vi "Create RC Connection Monitor.vi"(8 "error in (no error)":errorcluster, 10 "Configure":T1, 11 "RemoteControl in":refnum<class "RemoteControl.v2.lvclass">) -> (0 "error out":errorcluster, 3 "RemoteControl out":refnum<class "RemoteControl.v2.lvclass">)   [LabVIEW 2016, in "RemoteControl.v2.lvclass"]
uses:
  RemoteControl.v2.lvclass
  C:/Program Files (x86)/National Instruments/LabVIEW 2016/vi.lib/JKI/JKI SMO/SMO/SMO.lvclass
  Typedefs/PrivateEvents--RemoteControl.Configure.ctl
  Typedefs/RC Process Type--Enum.ctl
  RemoteControl.v2.lvclass/RemoteControl.v2.ctl
  <vilib>/JKI/JKI SMO/SMO/SMO.lvclass
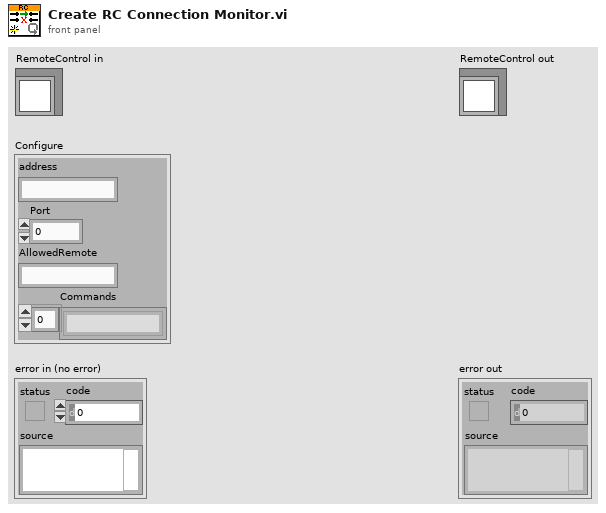
[diagram p1: front panel]
types:
  T1 = typedef "RemoteControl.v2.lvclass/PrivateEvents--RemoteControl.Configure.ctl" = cluster{"address":string, "Port":u16, "AllowedRemote":string, "Commands":string[]}
  T2 = typedef "RemoteControl.v2.lvclass/RC Process Type--Enum.ctl" = enum16{"Connection Monitor", "Server", "Client"}
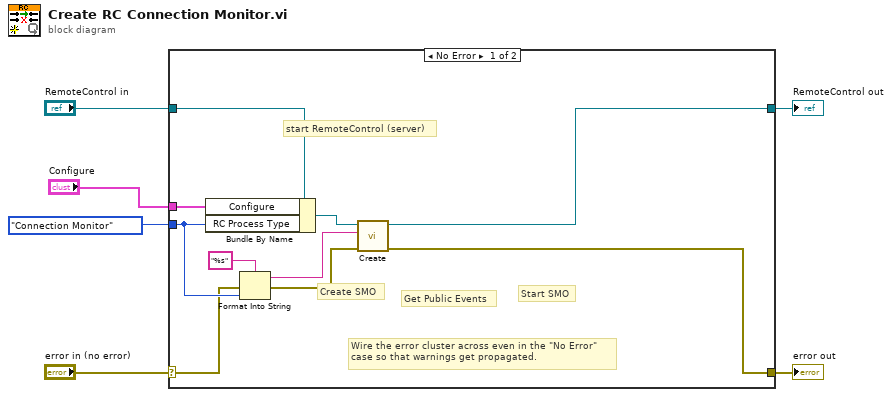
[diagram p0: block diagram]
diagram:
  n1 = case shown="No Error" "error in (no error)" {
    selector: "error in (no error)" -> [w9 w18]
    tunnel: [w8 w18] -> w5
    tunnel: [w7 w17] -> w3
    tunnel: "RemoteControl in" -> [w15 w17]
    tunnel: RC_Process_Type--Enum."Connection Monitor" ("RC Process Type") -> [w13 _]
    tunnel: "Configure" -> [w14 _]
    frame No Error {
      # "start RemoteControl (server)"
      # "Get Public Events"
      # "Start SMO"
      # "Create SMO"
      # "Wire the error cluster across even in the \"No Error\"\ncase so that warnings get propagated."
      n2 = Bundle By Name(cluster=w15, "Configure"=w14, "RC Process Type"=w13) -> (w16:refnum<class "RemoteControl.v2.lvclass">)
      n3 = Format Into String(format string="%s", error in=w9, w13) -> (resulting string=w11:string, error out=w10:errorcluster)  [unwired: 1 in]
      n4 = call <vilib>:"Create.vi"("error in (no error)"=w10, "Subsystem Name (optional)"=w11, "SMO"=w16) -> ("error out"=w8:errorcluster, "SMO out"=w7:refnum<class "RemoteControl.v2.lvclass">)  [unwired: 6 in, 1 out]
    }
    frame Error {
    }
  }
  "error out" <- w5
  "RemoteControl out" <- w3
